vi "Wait.vi"(8 "error in (no error)":errorcluster, 11 "Refnum in":T1) -> (0 "error out":errorcluster, 3 "Refnum out":T1)   [LabVIEW 2019, in "HD44780.lvlib"]
uses:
  HD44780.lvlib
  FPGA VI Reference.ctl
  <vilib>/rvi/interface/nirviReadWriteControl/nirviReadWriteControl.xnode
  NiFpgaLv.dll
  <vilib>/Utility/error.llb/Error Cluster From Error Code.vi
  <vilib>/rvi/interface/Simulation/niFpgaSimulationCallBeginRW.vi
  <vilib>/rvi/errors/niLvFpgaAdjustHostInterfaceError.vi
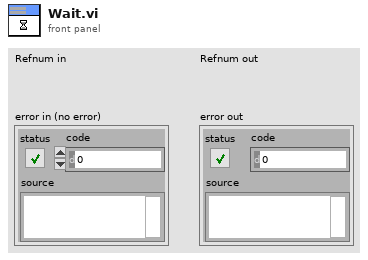
[diagram p1: front panel]
types:
  T1 = typedef "FPGA VI Reference.ctl" = refnum<k20>
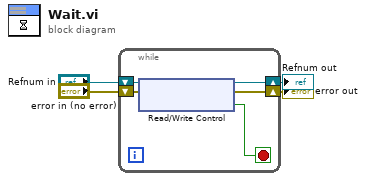
[diagram p0: block diagram]
diagram:
  n1 = while {
    shift-right: [w6] -> w4
    shift-left: "Refnum in" -> [w9]
    shift-right: [w7] -> w3
    shift-left: "error in (no error)" -> [w8]
    stop <- w5 stop-if-true
    n2 = xnode "Read/Write Control"("FPGA VI Reference In"=w9, "error in"=w8) -> ("FPGA VI Reference Out"=w6:T1, "error out"=w7:errorcluster, "Cmd Executed"=w5:bool)
  }
  "Refnum out" <- w4
  "error out" <- w3
